vi "U75.vi"() -> ()   [LabVIEW 2024]
uses:
  <vilib>/Instr/_visa.llb/VISA Configure Serial Port (Instr).vi
panel:
  out "Reponse":string
  out "Boolean":bool
  in  "Cancel Button":bool
  in  "stop":bool
  in  "OK Button":bool
  out "Array":dbl[](array[numeric])
  in  "error in (no error)":errorcluster
  in  "VISA resource name":refnum<visa-resource-name>
  out "XY Graph":cluster{"X":dbl, "Y":dbl}[](graph)
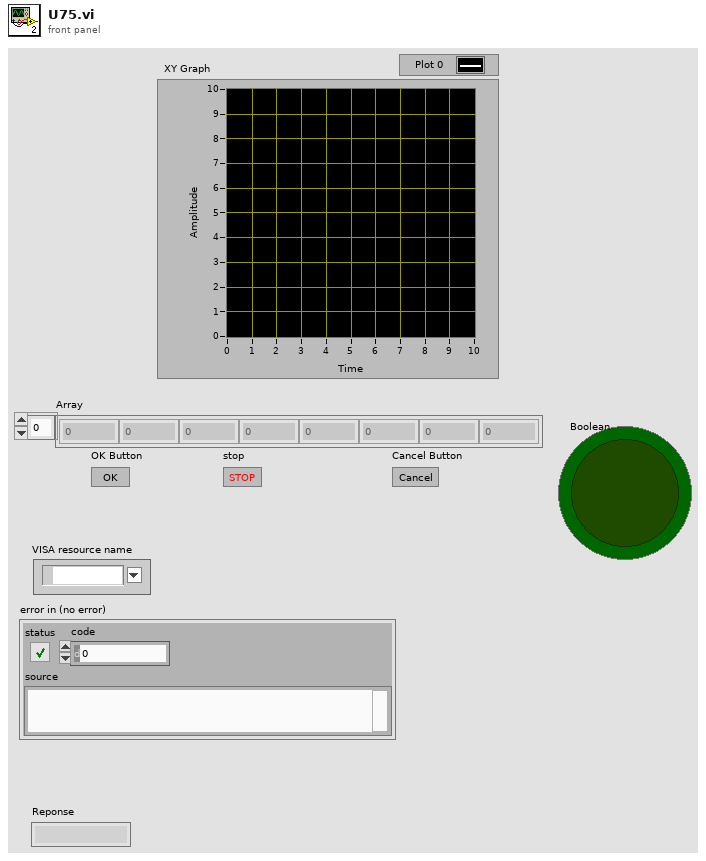
[diagram p1: front panel]
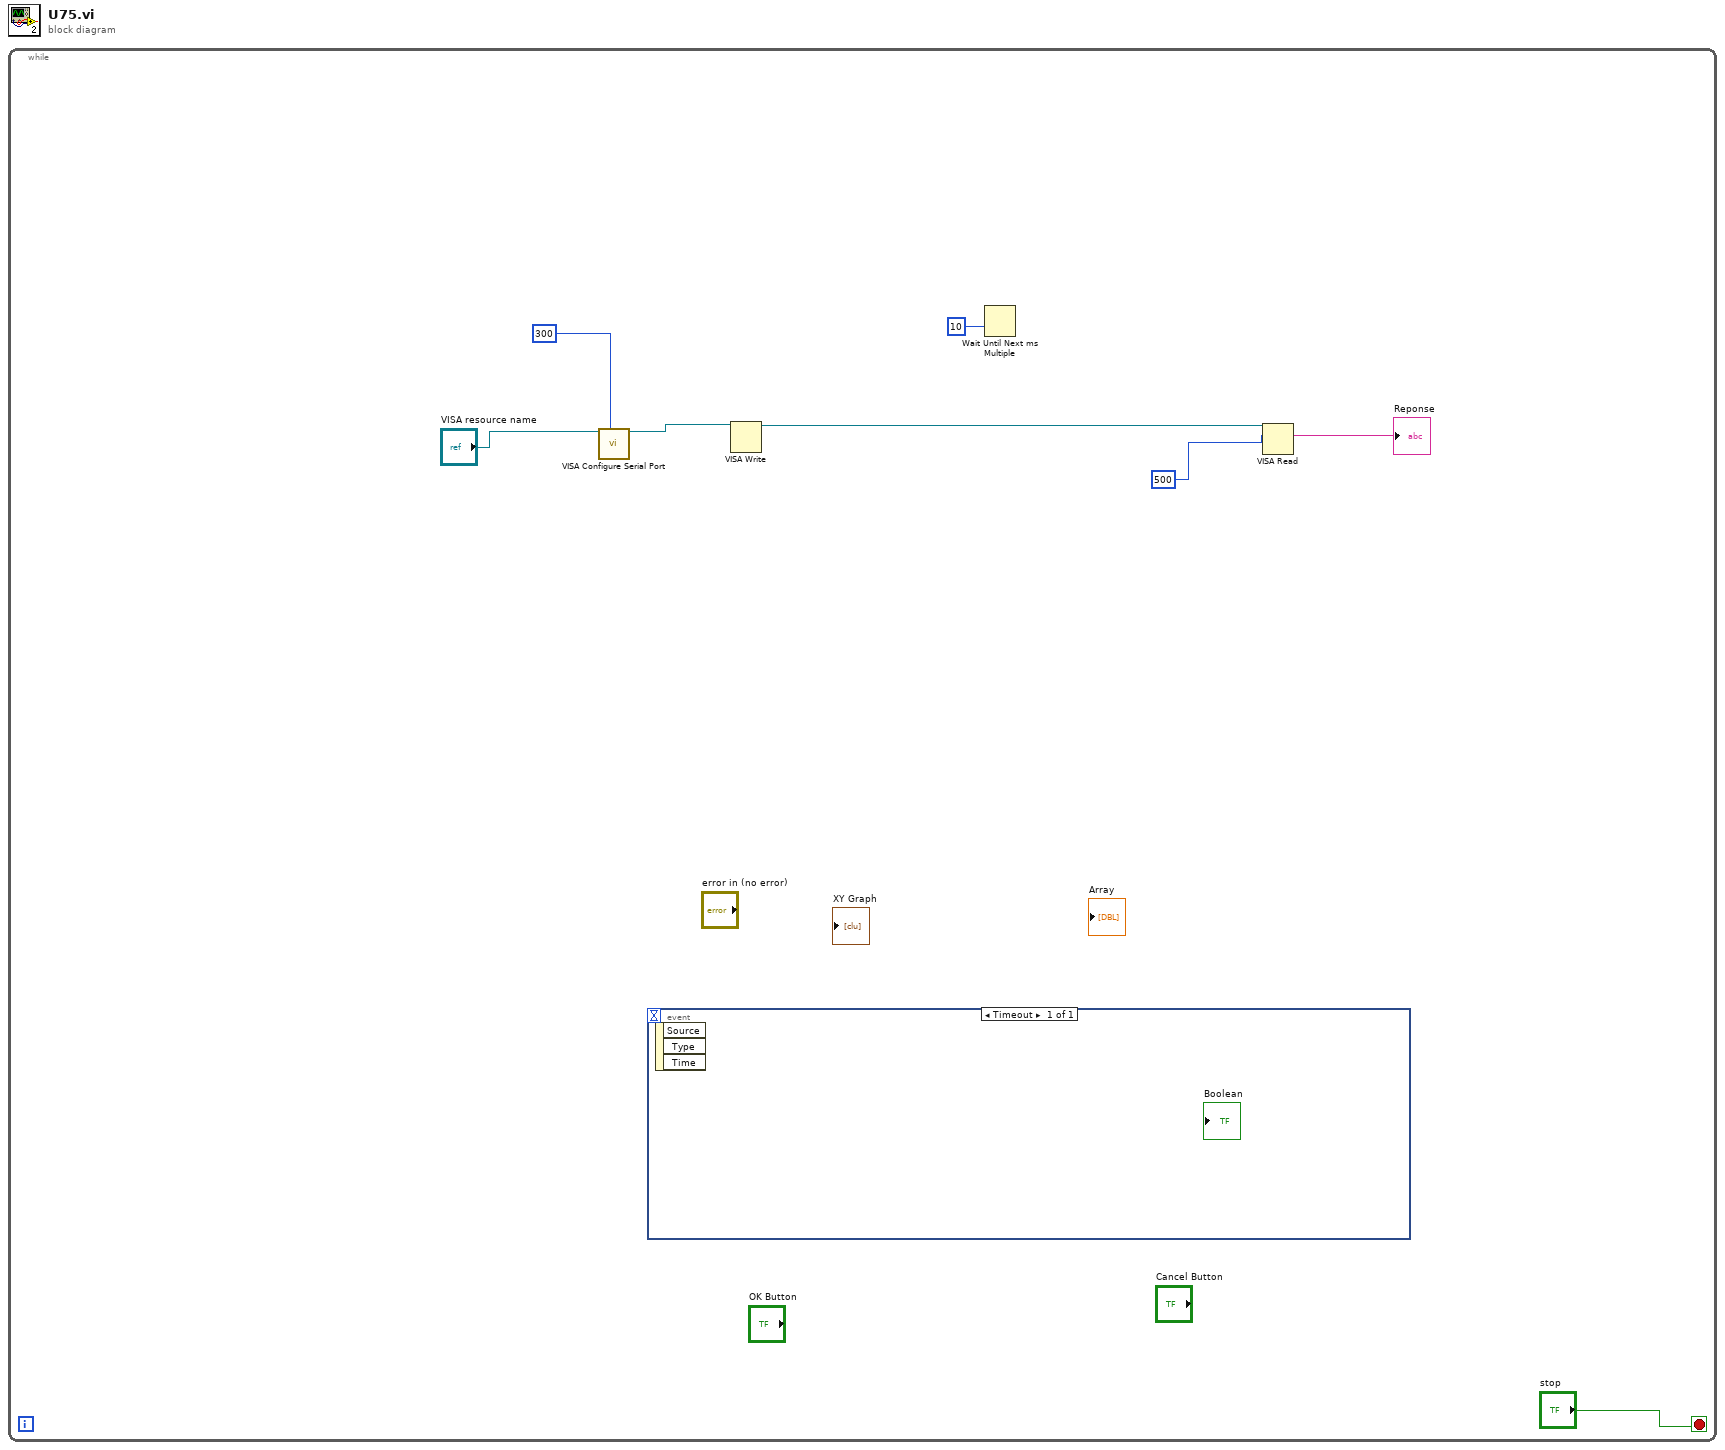
[diagram p0: block diagram]
diagram:
  n1 = while {
    stop <- "stop" stop-if-true
    n2 = call-poly "VISA Configure Serial Port"("VISA resource name"="VISA resource name", "timeout (10sec)"=300) -> ("VISA resource name out"=w2:refnum<visa-resource-name>)  [unwired: 12 in, 1 out]
    n3 = event shown="[0] Timeout" {
      selector: _ -> [_]
      dyn-events: _ -> [_]
      timeout: _ -> [_]
      event Timeout {
        n4 = event-data() -> ()  [unwired: 1 in, 3 out]
      }
    }
    n5 = VISA Write(VISA resource name=w2) -> (VISA resource name out=w1:refnum<visa-resource-name>)  [unwired: 2 in, 2 out]
    n6 = Wait Until Next ms Multiple(millisecond multiple=10) -> ()  [unwired: 1 out]
    n7 = VISA Read(VISA resource name=w1, byte count=500) -> (read buffer=→"Reponse":string)  [unwired: 1 in, 3 out]
  }
